vi "Input_4ch_v00.vi"(11 "Control":T7={"PII In 1"={"Lock"=FALSE, "Hold"=FALSE, "P Gain"=0, "P BS"=-5, "I Gain"=0, "I BS"=-10, "I2 G"=0, "I2 BS"=-26, "Scan Amp"=0, "Scan Off"=0, "Scan FS"=0, "SFS BS"=0, "I Max value"=10000, "I2 Max value"=10000, "Scope.Offset"=0, "Trigger Direction"=enum."either", "Scan-PII thresh"=0}, "PII In 2"={"Lock"=FALSE, "Hold"=FALSE, "P Gain"=0, "P BS"=-10, "I Gain"=0, "I BS"=-10, "I2 G"=0, "I2 BS"=-26, "Scan Amp"=0, "Scan Off"=0, "Scan FS"=0, "SFS BS"=0, "I Max value"=10000, "I2 Max value"=10000, "Scope.Offset"=0, "Trigger Direction"=enum."either", "Scan-PII thresh"=0}, "PII In 3"={"Lock"=FALSE, "Hold"=FALSE, "P Gain"=0, "P BS"=-10, "I Gain"=0, "I BS"=-10, "I2 G"=0, "I2 BS"=-26, "Scan Amp"=0, "Scan Off"=0, "Scan FS"=0, "SFS BS"=0, "I Max value"=10000, "I2 Max value"=10000, "Scope.Offset"=0, "Trigger Direction"=enum."either", "Scan-PII thresh"=0}, "Error scale"={"Pre-Offset"={"Pre-Offset 1"=2, "Pre-Offset 2"=0, "Pre-Offset 3"=0, "Pre-Offset 4"=0, "Pre-Offset 5"=2, "Pre-Offset 6"=0, "Pre-Offset 7"=2}, "Post-Offset "={"Offset 1"=0, "Offset 2"=300, "Offset 3"=0, "Offset 4"=0, "Offset 5"=0, "Offset 6"=0, "Offset 7"=0}, "Gains"={"Gain 1"=0, "Gain 2"=300, "Gain 3"=0, "Gain 4"=0, "Gain 5"=0, "Gain 6"=0, "Gain 7"=0}, "Bit Shifts"={"Bit Shift 1"=0, "Bit Shift 2"=300, "Bit Shift 3"=0, "Bit Shift 4"=0, "Bit Shift 5"=0, "Bit Shift 6"=0, "Bit Shift 7"=0}}, "Lock Thresh"={"EPR"=2, "HD A"=0, "HD B"=10, "HD C"=0}, "Re-Scan Thresh"={"EPR"=2, "HD A"=0, "HD B"=0, "HD C"=0}, "Theta"={"HD A Sin Theta"=0, "HD A Cos Theta"=0, "HD B Sin Theta"=0, "HD B Cos Theta"=0, "HD C Sin Theta"=0, "HD C Cos Theta"=0}, "Safety First"={"lim reset"=FALSE, "no limit"=FALSE, "pos slew rate * dt"=0, "neg slew rate * dt"=-10, "Hold All"=FALSE, "Count(Ticks)"=0}, "PII In 4"={"Lock"=FALSE, "Hold"=FALSE, "P Gain"=0, "P BS"=-10, "I Gain"=0, "I BS"=-10, "I2 G"=0, "I2 BS"=-26, "Scan Amp"=0, "Scan Off"=0, "Scan FS"=0, "SFS BS"=0, "I Max value"=10000, "I2 Max value"=10000, "Scope.Offset"=0, "Trigger Direction"=enum."either", "Scan-PII thresh"=0}}) -> (3 "Signals":T3={"PII In 1"={"Lock"=FALSE, "Hold"=FALSE, "P Gain"=0, "P BS"=0, "I Gain"=0, "I BS"=-10, "I2 G"=0, "I2 BS"=-26, "Scan Amp"=0, "Scan Off"=0, "Scan FS"=0, "SFS BS"=0, "I Max value"=10000, "I2 Max value"=10000, "Scope.Offset"=0, "Trigger Direction"=enum."either", "Scan-PII thresh"=0}, "PII In 2"={"Lock"=FALSE, "Hold"=FALSE, "P Gain"=0, "P BS"=0, "I Gain"=0, "I BS"=-10, "I2 G"=0, "I2 BS"=-26, "Scan Amp"=0, "Scan Off"=0, "Scan FS"=0, "SFS BS"=0, "I Max value"=10000, "I2 Max value"=10000, "Scope.Offset"=0, "Trigger Direction"=enum."either", "Scan-PII thresh"=0}, "PII In 3"={"Lock"=FALSE, "Hold"=FALSE, "P Gain"=0, "P BS"=0, "I Gain"=0, "I BS"=-10, "I2 G"=0, "I2 BS"=-26, "Scan Amp"=0, "Scan Off"=0, "Scan FS"=0, "SFS BS"=0, "I Max value"=10000, "I2 Max value"=10000, "Scope.Offset"=0, "Trigger Direction"=enum."either", "Scan-PII thresh"=0}, "Lock Thresh"={"EPR"=2, "HD A"=0, "HD B"=0, "HD C"=0}, "Re-Scan Thresh"={"EPR"=2, "HD A"=0, "HD B"=0, "HD C"=0}, "Safety First"={"lim reset"=FALSE, "no limit"=FALSE, "pos slew rate * dt"=0, "neg slew rate * dt"=-10, "Hold All"=FALSE, "Count(Ticks)"=4294967286}, "Graph Errors"={"EPR"=2, "HD A"=0, "HD B"=0, "HD C"=0}, "PII In 4"={"Lock"=FALSE, "Hold"=FALSE, "P Gain"=0, "P BS"=-10, "I Gain"=0, "I BS"=-10, "I2 G"=0, "I2 BS"=-26, "Scan Amp"=0, "Scan Off"=0, "Scan FS"=0, "SFS BS"=0, "I Max value"=10000, "I2 Max value"=10000, "Scope.Offset"=0, "Trigger Direction"=enum."either", "Scan-PII thresh"=0}}, 7 "HD Errors xp":T1)   [LabVIEW 2013]
doc: "Reads in and scales 8 inputs from the FPGA. For each homodyne lock 2 orthogonal error signals are combined in order to lock the local oscillator to an arbitrary phase."
uses:
  Strict Type Defs/FPGA Inputs 1SDI.ctl
  Strict Type Defs/Error Signals 1SDI.ctl
  Strict Type Defs/Control 1SDI Input.ctl
  Strict Type Defs/PII individual.ctl
  Strict Type Defs/Error Scale 1SDI.ctl
  Strict Type Defs/Lock Thresh 1SDI.ctl
  Strict Type Defs/Theta graph.ctl
  Strict Type Defs/Safety First.ctl
  Strict Type Defs/Signals 1SDI.ctl
  <vilib>/rvi/eio/common/nirviEmuTemplateMethod_errors.vi
  <vilib>/eio/EIONode/EIONode.xnode
panel:
  in  "x p Errors":T1={"HD A x"=0, "HD A p"=1800, "HD B x"=0, "HD B p"=0, "HD C p"=0, "HD C x"=0}
  out "Error Signals":T2={"EPR"=0, "HD A"=1800, "HD B"=0, "HD C"=0}
  in  "Signals":T3={"PII In 1"={"Lock"=FALSE, "Hold"=FALSE, "P Gain"=0, "P BS"=0, "I Gain"=0, "I BS"=-10, "I2 G"=0, "I2 BS"=-26, "Scan Amp"=0, "Scan Off"=0, "Scan FS"=0, "SFS BS"=0, "I Max value"=10000, "I2 Max value"=10000, "Scope.Offset"=0, "Trigger Direction"=enum."either", "Scan-PII thresh"=0}, "PII In 2"={"Lock"=FALSE, "Hold"=FALSE, "P Gain"=0, "P BS"=0, "I Gain"=0, "I BS"=-10, "I2 G"=0, "I2 BS"=-26, "Scan Amp"=0, "Scan Off"=0, "Scan FS"=0, "SFS BS"=0, "I Max value"=10000, "I2 Max value"=10000, "Scope.Offset"=0, "Trigger Direction"=enum."either", "Scan-PII thresh"=0}, "PII In 3"={"Lock"=FALSE, "Hold"=FALSE, "P Gain"=0, "P BS"=0, "I Gain"=0, "I BS"=-10, "I2 G"=0, "I2 BS"=-26, "Scan Amp"=0, "Scan Off"=0, "Scan FS"=0, "SFS BS"=0, "I Max value"=10000, "I2 Max value"=10000, "Scope.Offset"=0, "Trigger Direction"=enum."either", "Scan-PII thresh"=0}, "Lock Thresh"={"EPR"=2, "HD A"=0, "HD B"=0, "HD C"=0}, "Re-Scan Thresh"={"EPR"=2, "HD A"=0, "HD B"=0, "HD C"=0}, "Safety First"={"lim reset"=FALSE, "no limit"=FALSE, "pos slew rate * dt"=0, "neg slew rate * dt"=-10, "Hold All"=FALSE, "Count(Ticks)"=4294967286}, "Graph Errors"={"EPR"=2, "HD A"=0, "HD B"=0, "HD C"=0}, "PII In 4"={"Lock"=FALSE, "Hold"=FALSE, "P Gain"=0, "P BS"=-10, "I Gain"=0, "I BS"=-10, "I2 G"=0, "I2 BS"=-26, "Scan Amp"=0, "Scan Off"=0, "Scan FS"=0, "SFS BS"=0, "I Max value"=10000, "I2 Max value"=10000, "Scope.Offset"=0, "Trigger Direction"=enum."either", "Scan-PII thresh"=0}}
  in  "Error Signals":T2
  in  "FPGA Inputs":T10
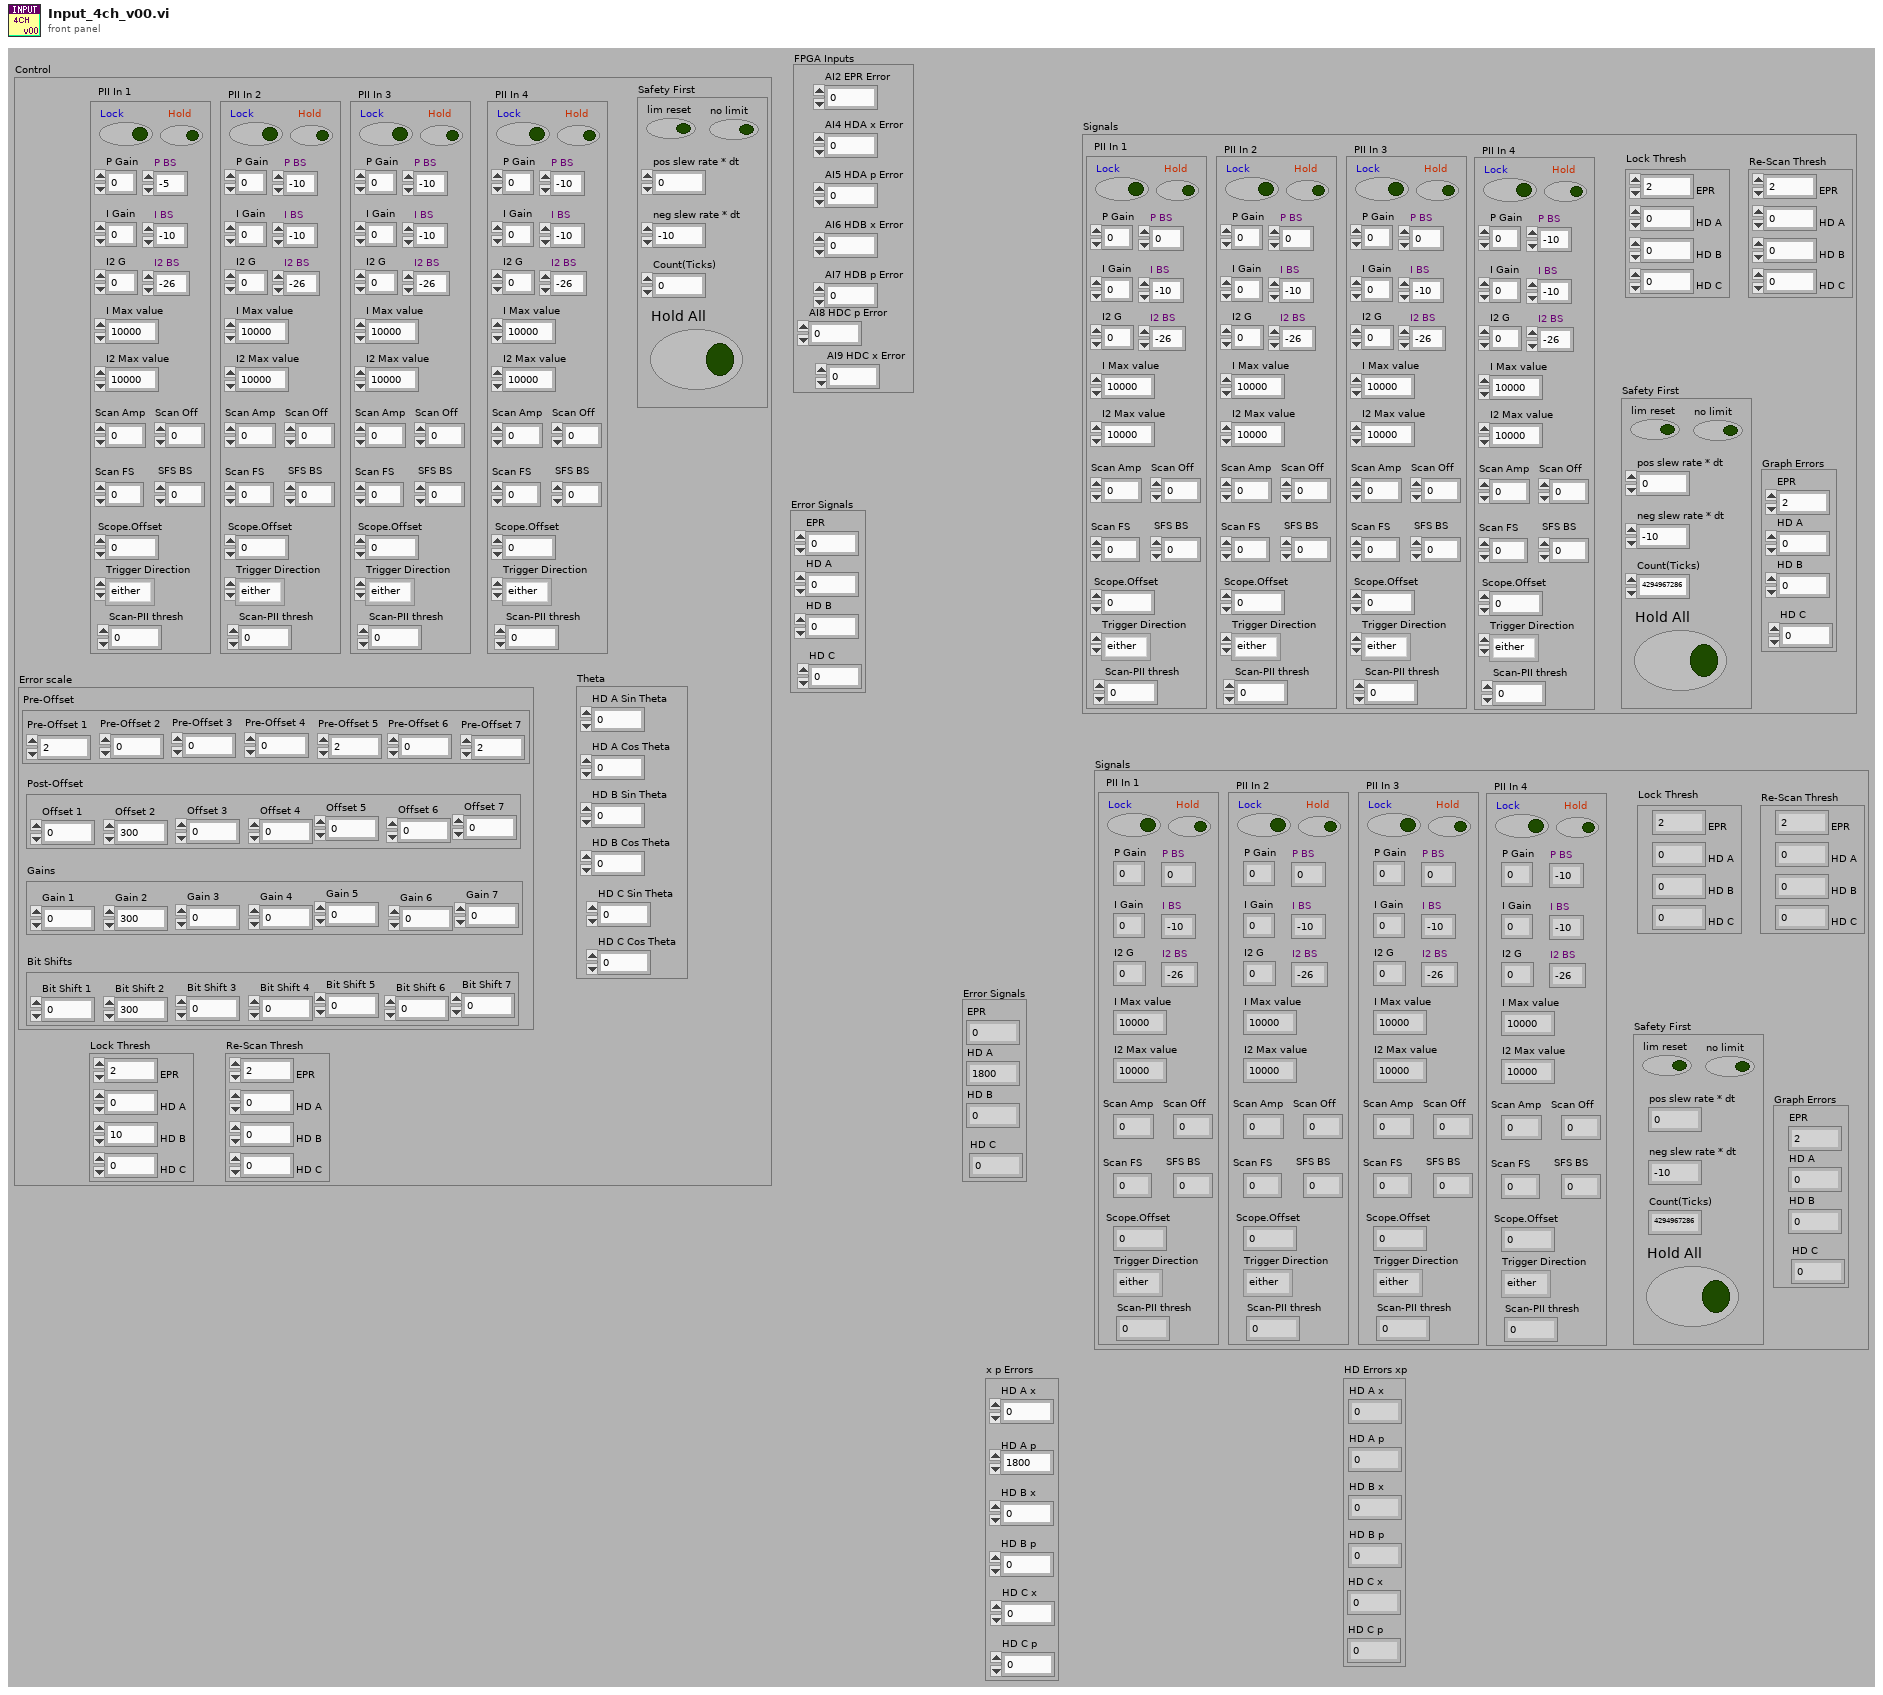
[diagram p1: front panel]
types:
  T1 = cluster{"HD A x":i16, "HD A p":i16, "HD B x":i16, "HD B p":i16, "HD C p":i16, "HD C x":i16}
  T2 = typedef "Error Signals 1SDI.ctl" = cluster{"EPR":i16, "HD A":i16, "HD B":i16, "HD C":i16}
  T3 = typedef "Signals 1SDI.ctl" = cluster{"PII In 1":T4, "PII In 2":T4, "PII In 3":T4, "Lock Thresh":T5, "Re-Scan Thresh":T5, "Safety First":T6, "Graph Errors":T2, "PII In 4":T4}
  T4 = typedef "PII individual.ctl" = cluster{"Lock":bool, "Hold":bool, "P Gain":i32, "P BS":i16, "I Gain":i32, "I BS":i16, "I2 G":i32, "I2 BS":i16, "Scan Amp":i16, "Scan Off":i16, "Scan FS":u16, "SFS BS":i16, "I Max value":i32, "I2 Max value":i32, "Scope.Offset":i16, "Trigger Direction":enum8{"either", "minus-plus", "plus-minus"}, "Scan-PII thresh":i16}
  T5 = typedef "Lock Thresh 1SDI.ctl" = cluster{"EPR":i16, "HD A":i16, "HD B":i16, "HD C":i16}
  T6 = typedef "Safety First.ctl" = cluster{"lim reset":bool, "no limit":bool, "pos slew rate * dt":i16, "neg slew rate * dt":i16, "Hold All":bool, "Count(Ticks)":u32}
  T7 = typedef "Control 1SDI Input.ctl" = cluster{"PII In 1":T4, "PII In 2":T4, "PII In 3":T4, "Error scale":T8, "Lock Thresh":T5, "Re-Scan Thresh":T5, "Theta":T9, "Safety First":T6, "PII In 4":T4}
  T8 = typedef "Error Scale 1SDI.ctl" = cluster{"Pre-Offset":cluster{"Pre-Offset 1":i16, "Pre-Offset 2":i16, "Pre-Offset 3":i16, "Pre-Offset 4":i16, "Pre-Offset 5":i16, "Pre-Offset 6":i16, "Pre-Offset 7":i16}, "Post-Offset ":cluster{"Offset 1":i16, "Offset 2":i16, "Offset 3":i16, "Offset 4":i16, "Offset 5":i16, "Offset 6":i16, "Offset 7":i16}, "Gains":cluster{"Gain 1":i16, "Gain 2":i16, "Gain 3":i16, "Gain 4":i16, "Gain 5":i16, "Gain 6":i16, "Gain 7":i16}, "Bit Shifts":cluster{"Bit Shift 1":i16, "Bit Shift 2":i16, "Bit Shift 3":i16, "Bit Shift 4":i16, "Bit Shift 5":i16, "Bit Shift 6":i16, "Bit Shift 7":i16}}
  T9 = typedef "Theta graph.ctl" = cluster{"HD A Sin Theta":i32, "HD A Cos Theta":i32, "HD B Sin Theta":i32, "HD B Cos Theta":i32, "HD C Sin Theta":i32, "HD C Cos Theta":i32}
  T10 = typedef "FPGA Inputs 1SDI.ctl" = cluster{"AI2 EPR Error":i16, "AI4 HDA x Error":i16, "AI5 HDA p Error":i16, "AI6 HDB x Error":i16, "AI7 HDB p Error":i16, "AI8 HDC p Error":i16, "AI9 HDC x Error":i16}
  T11 = cluster{"Offset 1":i16, "Offset 2":i16, "Offset 3":i16, "Offset 4":i16, "Offset 5":i16, "Offset 6":i16, "Offset 7":i16}
  T12 = cluster{"Bit Shift 1":i16, "Bit Shift 2":i16, "Bit Shift 3":i16, "Bit Shift 4":i16, "Bit Shift 5":i16, "Bit Shift 6":i16, "Bit Shift 7":i16}
  T13 = cluster{"Gain 1":i16, "Gain 2":i16, "Gain 3":i16, "Gain 4":i16, "Gain 5":i16, "Gain 6":i16, "Gain 7":i16}
  T14 = cluster{"Pre-Offset 1":i16, "Pre-Offset 2":i16, "Pre-Offset 3":i16, "Pre-Offset 4":i16, "Pre-Offset 5":i16, "Pre-Offset 6":i16, "Pre-Offset 7":i16}
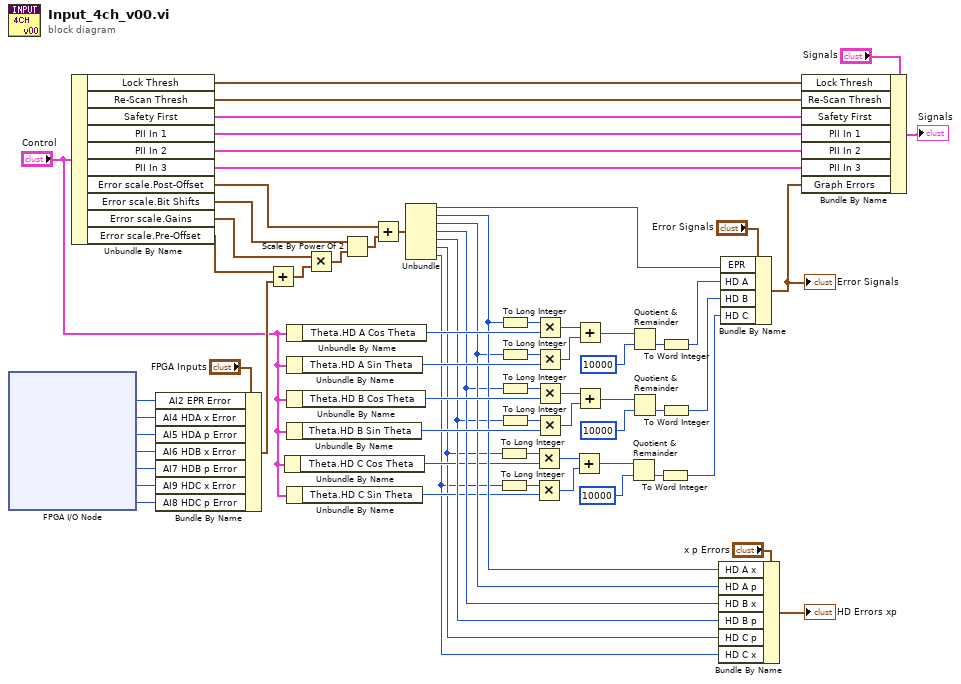
[diagram p0: block diagram]
diagram:
  n1 = xnode "FPGA I/O Node"() -> ("Connector0/AI0"=w25:i16, "Connector0/AI1"=w24:i16, "Connector0/AI2"=w23:i16, "Connector0/AI3"=w22:i16, "Connector0/AI4"=w21:i16, "Connector0/AI5"=w6:i16, "Connector0/AI6"=w5:i16)  [unwired: 7 in, 7 out]
  n2 = Unbundle By Name("Control") -> ("Lock Thresh"=w37:T5, "Re-Scan Thresh"=w36:T5, "Safety First"=w38:T6, "PII In 1"=w59:T4, "PII In 2"=w58:T4, "PII In 3"=w57:T4, "Error scale.Post-Offset"=w67:T11, "Error scale.Bit Shifts"=w27:T12, "Error scale.Gains"=w64:T13, "Error scale.Pre-Offset"=w65:T14)
  n3 = Bundle By Name(cluster="FPGA Inputs", "AI2 EPR Error"=w25, "AI4 HDA x Error"=w24, "AI5 HDA p Error"=w23, "AI6 HDB x Error"=w22, "AI7 HDB p Error"=w21, "AI9 HDC x Error"=w6, "AI8 HDC p Error"=w5) -> (w56:T10)
  n4 = Add(x=w65, y=w56) -> (x+y=w66:T10)
  n5 = Unbundle By Name("Control") -> ("Theta.HD C Cos Theta"=w4:i32)
  n6 = Unbundle By Name("Control") -> ("Theta.HD A Cos Theta"=w53:i32)
  n7 = Unbundle By Name("Control") -> ("Theta.HD A Sin Theta"=w49:i32)
  n8 = Unbundle By Name("Control") -> ("Theta.HD B Cos Theta"=w42:i32)
  n9 = Unbundle By Name("Control") -> ("Theta.HD B Sin Theta"=w46:i32)
  n10 = Unbundle By Name("Control") -> ("Theta.HD C Sin Theta"=w3:i32)
  n11 = Multiply(x=w64, y=w66) -> (x*y=w29:T10)
  n12 = Scale By Power Of 2(n=w27, x=w29) -> (x*2^n=w28:T10)
  n13 = Add(x=w67, y=w28) -> (x+y=w26:T10)
  n14 = Unbundle(w26) -> ("AI2 EPR Error"=w20:i16, "AI4 HDA x Error"=w19:i16, "AI5 HDA p Error"=w18:i16, "AI6 HDB x Error"=w17:i16, "AI7 HDB p Error"=w16:i16, "AI8 HDC p Error"=w2:i16, "AI9 HDC x Error"=w1:i16)
  n15 = To Long Integer(number=w2) -> (32bit integer=w12:i32)
  n16 = To Long Integer(number=w1) -> (32bit integer=w14:i32)
  n17 = To Long Integer(number=w19) -> (32bit integer=w54:i32)
  n18 = To Long Integer(number=w18) -> (32bit integer=w50:i32)
  n19 = To Long Integer(number=w17) -> (32bit integer=w41:i32)
  n20 = To Long Integer(number=w16) -> (32bit integer=w45:i32)
  n21 = Multiply(x=w12, y=w4) -> (x*y=w13:i32)
  n22 = Multiply(x=w14, y=w3) -> (x*y=w9:i32)
  n23 = Multiply(x=w54, y=w53) -> (x*y=w52:i32)
  n24 = Multiply(x=w50, y=w49) -> (x*y=w48:i32)
  n25 = Multiply(x=w41, y=w42) -> (x*y=w43:i32)
  n26 = Multiply(x=w45, y=w46) -> (x*y=w47:i32)
  n27 = Add(x=w13, y=w9) -> (x+y=w8:i32)
  n28 = Add(x=w52, y=w48) -> (x+y=w51:i32)
  n29 = Add(x=w43, y=w47) -> (x+y=w44:i32)
  n30 = Quotient & Remainder(x=w8, y=10000) -> (floor(x/y)=w11:i32)  [unwired: 1 out]
  n31 = Quotient & Remainder(x=w51, y=10000) -> (floor(x/y)=w33:i32)  [unwired: 1 out]
  n32 = Quotient & Remainder(x=w44, y=10000) -> (floor(x/y)=w35:i32)  [unwired: 1 out]
  n33 = To Word Integer(number=w11) -> (16bit integer=w7:i16)
  n34 = To Word Integer(number=w33) -> (16bit integer=w32:i16)
  n35 = To Word Integer(number=w35) -> (16bit integer=w34:i16)
  n36 = Bundle By Name(cluster="x p Errors", "HD A x"=w19, "HD A p"=w18, "HD B x"=w17, "HD B p"=w16, "HD C p"=w2, "HD C x"=w1) -> (→"HD Errors xp":T1)
  n37 = Bundle By Name(cluster="Error Signals", "EPR"=w20, "HD A"=w32, "HD B"=w34, "HD C"=w7) -> (w39:T2)
  "Error Signals" <- w39
  n38 = Bundle By Name(cluster="Signals", "Lock Thresh"=w37, "Re-Scan Thresh"=w36, "Safety First"=w38, "PII In 1"=w59, "PII In 2"=w58, "PII In 3"=w57, "Graph Errors"=w39) -> (→"Signals":T3)
